vi "Set Angle Motor.vi"(9 "Hold":bool, 11 "Motor Speed":dbl) -> ()   [LabVIEW 2012]
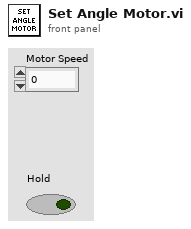
[diagram p1: front panel]
types:
  T1 = typedef "WPI_DigitalInputDevRef.ctl" = cluster{"DevStatus":errorcluster, "DIO Channel":T2, "Digital Module":T3}
  T2 = typedef "FPGA_DIOChannel.ctl" = enum8{"DIO 1", "DIO 2", "DIO 3", "DIO 4", "DIO 5", "DIO 6", "DIO 7", "DIO 8", "DIO 9", "DIO 10", "DIO 11", "DIO 12", "DIO 13", "DIO 14", "Invalid"}
  T3 = typedef "FPGA_TypedefDigitalModule.ctl" = enum16{"Digital Module 1", "Digital Module 2"}
  T4 = typedef "WPI_MotorControlDeviceRef.ctl" = cluster{"DeviceStatus":errorcluster, "Type":enum16{"PWM", "CAN"}, "PWM":cluster{"Digital Module":T3, "PWM Channel":T5, "DeadBand":T6}, "CAN":cluster{"Device Number":u8, "Control Mode":T7, "Semaphore":T8, "Max Vout":dbl}, "Invert":bool, "TransformRef":T9, "InvTransformRef":T9}
  T5 = typedef "FPGA_DIOPWMChannel.ctl" = enum8{"PWM 1", "PWM 2", "PWM 3", "PWM 4", "PWM 5", "PWM 6", "PWM 7", "PWM 8", "PWM 9", "PWM 10", "Invalid"}
  T6 = typedef "WPI_PWMDeadband.ctl" = cluster{"Name":string, "maxPositivePwm":i32, "minPositivePwm":i32, "centerPwm":i32, "maxNegativePwm":i32, "minNegativePwm":i32, "angularRange":u16}
  T7 = typedef "WPI_CANJaguar_ControlMode.ctl" = enum8{"Percent VBus", "Current", "Speed", "Position", "Voltage"}
  T8 = typedef "Semaphore RefNum" = refnum<k1>
  T9 = typedef "WPI_PWMTransform_ConPane.ctl" = refnum<vi>
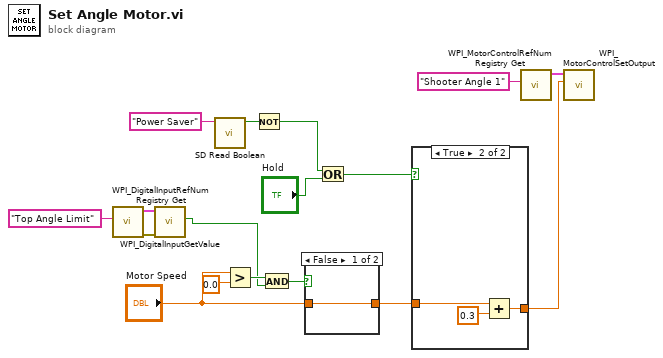
[diagram p0: block diagram]
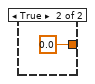
[diagram p3: hidden frame]
diagram:
  n1 = call <vilib>:"WPI_DigitalInputRefNum Registry Get.vi"("refnum name"="Top Angle Limit") -> ("error out"=w3:errorcluster, "DigitalInputDevRef"=w2:T1)  [unwired: 9 in]
  n2 = call <vilib>:"WPI_DigitalInputGetValue.vi"("error in (no error)"=w3, "DigitalInputDevRef"=w2) -> ("Value"=w1:bool)  [unwired: 7 in, 2 out]
  n3 = call <vilib>:"SD Read Boolean.vi"("Name"="Power Saver") -> ("Boolean"=w6:bool)  [unwired: 8 in, 2 out]
  n4 = Greater?(x="Motor Speed", y=0.0) -> (0:w12:bool)
  n5 = Not(x=w6) -> (.not. x?=w5:bool)
  n6 = And(x=w12, y=w1) -> (x .and. y?=w15:bool)
  n7 = case shown="False" w15 {
    tunnel: "Motor Speed" -> [w18 _]
    tunnel: [w18 0.0 ("Motor Speed")] -> w11
    frame False {
    }
    frame True {
    }
  }
  n8 = Or(x=w5, y="Hold") -> (x .or. y?=w7:bool)
  n9 = case shown="True" w7 {
    tunnel: w11 -> [w20 w22]
    tunnel: [w20 w21] -> w10
    frame False {
    }
    frame True {
      n10 = Add(x=w22, y=0.3) -> (x+y=w21:dbl)
    }
  }
  n11 = call <vilib>:"WPI_MotorControlRefNum Registry Get.vi"("refnum name"="Shooter Angle 1") -> ("MotorControlDevRef"=w16:T4)  [unwired: 9 in, 1 out]
  n12 = call <vilib>:"WPI_MotorControlSetOutput.vi"("Output"=w10, "MotorControlDevRef"=w16) -> ()  [unwired: 7 in, 3 out]
